vi "IRSweep.vi"() -> ()   [LabVIEW 2014]
uses:
  <vilib>/Utility/file.llb/Write To Spreadsheet File (DBL).vi
panel:
  in  "file path":path
  out "Position":i32
  in  "Stop":bool
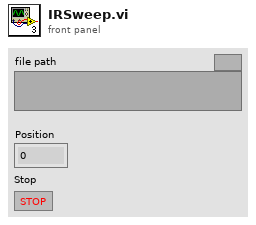
[diagram p1: front panel]
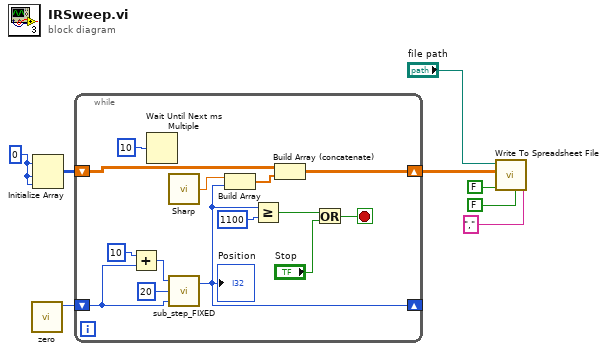
[diagram p0: block diagram]
diagram:
  w8 = 0
  n1 = call "zero.vi"() -> ("PositionOut"=w6:i32)  [unwired: 11 in]
  n2 = Initialize Array(w8, w8, w8) -> (w7:i32[][])
  n3 = while {
    shift-right: [w12] -> _
    shift-left: w6 -> [w10]
    shift-right: [w13] -> w1
    shift-left: w7 -> [w20]
    stop <- w17 stop-if-true
    n4 = Add(x=10, y=w10) -> (x+y=w11:i32)
    n5 = Wait Until Next ms Multiple(millisecond multiple=u32 10) -> ()  [unwired: 1 out]
    n6 = call "Sharp.vi"() -> ("Slide 2"=w18:dbl)
    n7 = call "sub_step_FIXED.vi"("Current Position"=w10, "millisecond multiple"=u32 20, "Desired Position"=w11) -> ("Position Out"=w12:i32)  [unwired: 1 in]
    "Position" <- w12
    n8 = Build Array(w18, w12) -> (w19:dbl[])
    n9 = Greater Or Equal?(x=w12, y=1100) -> (x >= y?=w15:bool)
    n10 = Build Array (concatenate)(w20, w19) -> (w13:dbl[][])
    n11 = Or(x=w15, y="Stop") -> (x .or. y?=w17:bool)
  }
  n12 = call-poly <vilib>:"Write To Spreadsheet File.vi"("delimiter (\\t)"="," ("delimiter (\\t)"), "transpose? (no:F)"=FALSE, "append to file? (new file:F)"=FALSE, "2D data"=w1, "file path (dialog if empty)"="file path") -> ()  [unwired: 3 in, 1 out]
